vi "Lockin-4461 IV mode trigger and wait.vi"(8 "error in (no error)":errorcluster, 11 "Channels: AO":T1={"AO amp (V)"=[1.0, 0.0, 0.0, 0.0, 0.0, 0.0, 0.0, 0.0], "AO DC (V)"=[0.0, 0.0, 0.0, 0.0, 0.0, 0.0, 0.0, 0.0], "AO f (Hz)"=[1.0, 1.0, 1.0, 1.0, 1.0, 1.0, 1.0, 1.0], "AO phi (deg)"=[0.0, 0.0, 0.0, 0.0, 0.0, 0.0, 0.0, 0.0], "function"=[enum."Triangle Wave", enum."Sine Wave", enum."Sine Wave", enum."Sine Wave", enum."Sine Wave", enum."Sine Wave", enum."Sine Wave", enum."Sine Wave"]} {"AO f (Hz)" min=0.001 max=10000.0; "AO DC (V)" format="%#_6p"; "AO amp (V)" format="%#_6p"}) -> (0 "error out":errorcluster)   [LabVIEW 2016]
uses:
  Typedefs/AO-cluster.ctl
  Typedefs/AO_Amp-array.ctl
  Typedefs/AO_DC-array.ctl
  Typedefs/AO_f-array.ctl
  Typedefs/AO_phi-array.ctl
  Typedefs/Function-array.ctl
  Typedefs/Function-enum.ctl
panel:
  in  "stop":bool
  out "timer (s)":dbl=1.2239999771118164
  # "This VI triggers the lockin and waits until the acquisition is complete"
  # "0"
  # "1"
  # "2"
  # "3"
  # "4"
  # "5"
  # "6"
  # "7"
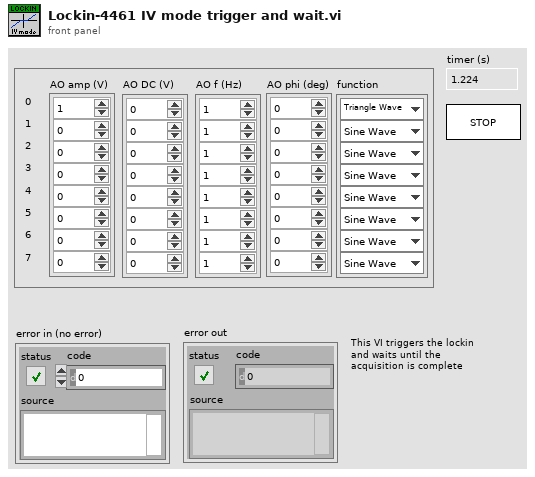
[diagram p1: front panel]
types:
  T1 = typedef "AO-cluster.ctl" = cluster{"AO amp (V)":T2, "AO DC (V)":T3, "AO f (Hz)":T4, "AO phi (deg)":T5, "function":T6}
  T2 = typedef "AO_Amp-array.ctl" = dbl[]
  T3 = typedef "AO_DC-array.ctl" = dbl[]
  T4 = typedef "AO_f-array.ctl" = dbl[]
  T5 = typedef "AO_phi-array.ctl" = dbl[]
  T6 = typedef "Function-array.ctl" = T7[]
  T7 = typedef "Function-enum.ctl" = enum16{"Sine Wave", "Triangle Wave", "Square Wave", "Sawtooth Wave"}
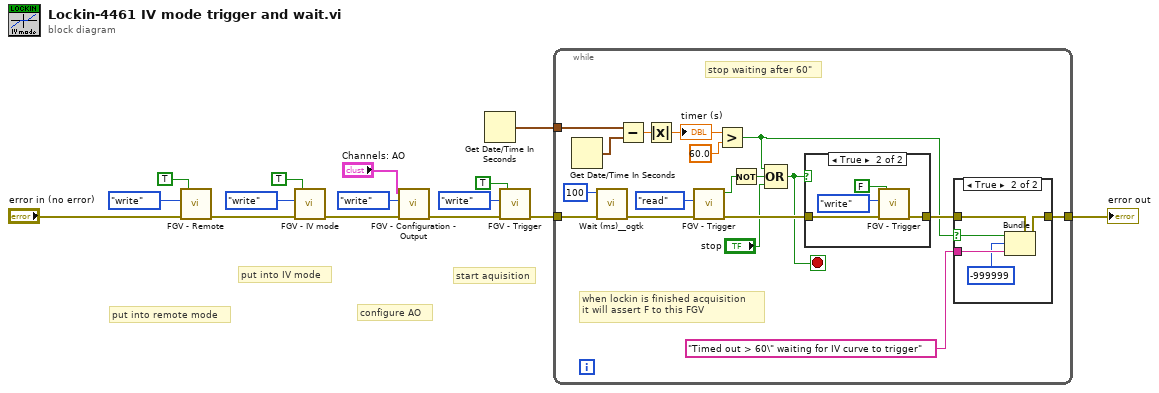
[diagram p0: block diagram]
diagram:
  # "start aquisition"
  # "configure AO"
  # "put into IV mode"
  # "put into remote mode"
  n1 = call "FGV - Remote.vi"("error in"="error in (no error)", "Function"=enum16{"write", "read"}."write", "Remote Mode"=TRUE ("Trigger")) -> ("error out"=w7:errorcluster)  [unwired: 3 in, 1 out]
  n2 = call "FGV - IV mode.vi"("error in"=w7, "Function"=enum16{"write", "read"}."write", "IV mode"=TRUE ("Trigger")) -> ("error out"=w4:errorcluster)  [unwired: 3 in, 1 out]
  n3 = call "FGV - Configuration - Output.vi"("error in"=w4, "Function"=enum16{"write", "read"}."write", "Channels: AO"="Channels: AO") -> ("error out"=w3:errorcluster)  [unwired: 3 in, 1 out]
  n4 = Get Date/Time In Seconds() -> (seconds since 1Jan1904=w12:timestamp)
  n5 = call "FGV - Trigger.vi"("error in"=w3, "Function"=enum16{"write", "read"}."write", "Trigger"=TRUE) -> ("error out"=w13:errorcluster)  [unwired: 3 in, 1 out]
  n6 = while {
    tunnel: w13 -> [w25]
    tunnel: w12 -> [w32]
    tunnel: [w29] -> w11
    stop <- w16 stop-if-true
    # "stop waiting after 60\""
    # "when lockin is finished acquisition\nit will assert F to this FGV"
    n7 = Get Date/Time In Seconds() -> (seconds since 1Jan1904=w22:timestamp)
    n8 = call <userlib>:"Wait (ms)__ogtk.vi"("error in (no error)"=w25, "milliseconds to wait"=u32 100) -> ("error out"=w24:errorcluster)  [unwired: 8 in, 1 out]
    n9 = Subtract(x=w32, y=w22) -> (x-y=w31:dbl)
    n10 = Absolute Value(x=w31) -> (abs(x)=w21:dbl)
    "timer (s)" <- w21
    n11 = call "FGV - Trigger.vi"("error in"=w24, "Function"=enum16{"write", "read"}."read") -> ("error out"=w28:errorcluster, "Trigger 2"=w19:bool)  [unwired: 4 in]
    n12 = Greater?(x=w21, y=60.0) -> (0:w20:bool)
    n13 = Not(x=w19) -> (.not. x?=w18:bool)
    n14 = Compound Arithmetic op=OR(w20, w18, "stop") -> (w16:bool)
    n15 = case shown="True" w16 {
      tunnel: w28 -> [w34 w36]
      tunnel: [w34 w35] -> w27
      frame False {
      }
      frame True {
        n16 = call "FGV - Trigger.vi"("error in"=w36, "Function"=enum16{"write", "read"}."write", "Trigger"=FALSE) -> ("error out"=w35:errorcluster)  [unwired: 3 in, 1 out]
      }
    }
    n17 = case shown="True" w20 {
      selector: w20 -> [_ w42]
      tunnel: "Timed out > 60\" waiting for IV curve to trigger" ("source") -> [_ w44]
      tunnel: w27 -> [w39 w43]
      tunnel: [w39 w41] -> w29
      frame False {
      }
      frame True {
        n18 = Bundle(cluster=w43, "status"=w42, "code"=-999999, "source"=w44) -> (w41:errorcluster)
      }
    }
  }
  "error out" <- w11
